vi "Day 12 Task 1 no recurse.vi"() -> ()   [LabVIEW 2018]
uses:
  Cave Info1.ctl
  <userlib>/_OpenG.lib/array/array.llb/Remove Duplicates from 1D Array (String)__ogtk.vi
  <userlib>/_OpenG.lib/array/array.llb/Search 1D Array (String)__ogtk.vi
panel:
  out "size(s)":i32
  out "Valid paths found":cluster{"Path":string[]}[](array[cluster])
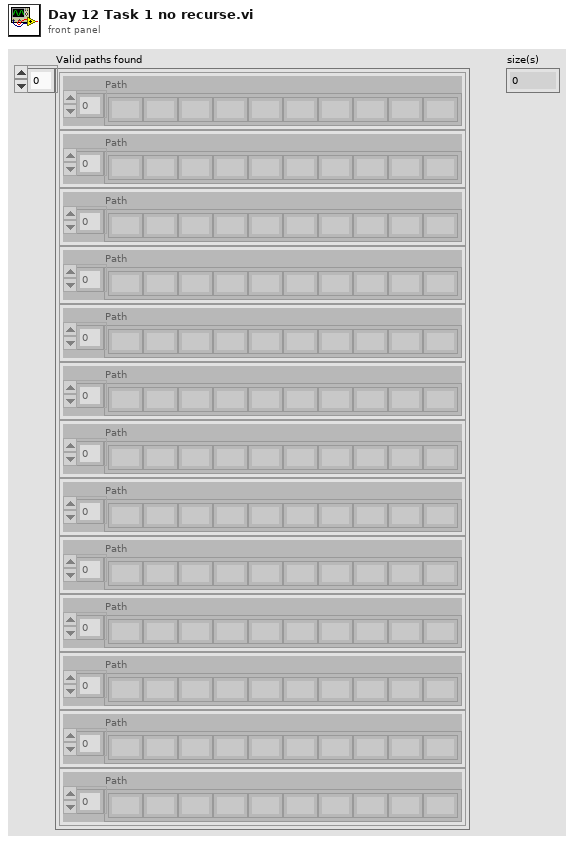
[diagram p1: front panel]
types:
  T1 = typedef "Cave Info1.ctl" = cluster{"Cave":string, "Is small?":bool, "Connections":string[]}
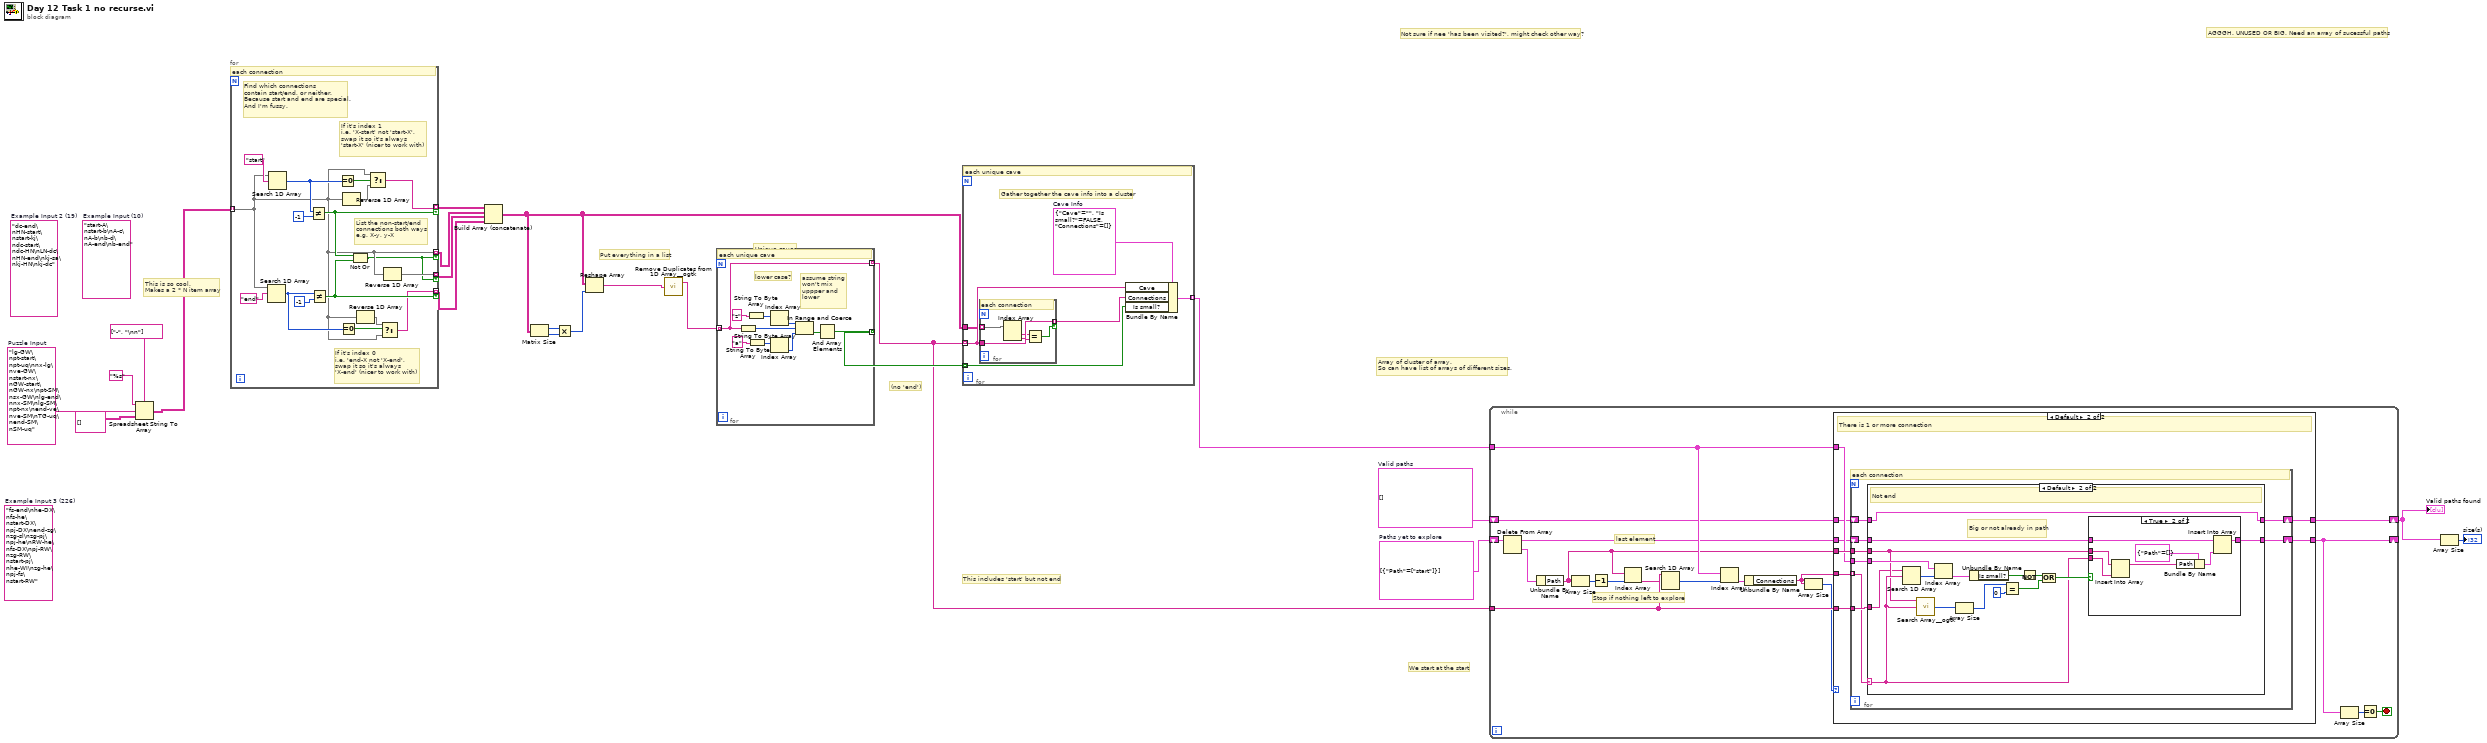
[diagram p0: block diagram]
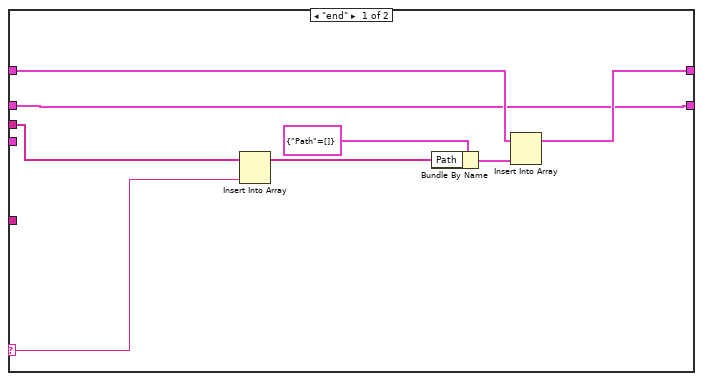
[diagram p3: hidden frame]
diagram:
  w7 = cluster{"Path":string[]}[] []  # Valid paths
  w9 = cluster{"Path":string[]}[] [{"Path"=["start"]}]  # Paths yet to explore
  (unwired) "fs-end\nhe-DX\nfs-he\nstart-DX\npj-DX\nend-zg\nzg-sl\nzg-pj\npj-he\nRW-he\nfs-DX\npj-RW\nzg-RW\nstart-pj\nhe-WI\nzg-he\npj-fs\nstart-RW"  # Example Input 3 (226)
  (unwired) "dc-end\nHN-start\nstart-kj\ndc-start\ndc-HN\nLN-dc\nHN-end\nkj-sa\nkj-HN\nkj-dc"  # Example Input 2 (19)
  w1 = "lg-GW\npt-start\npt-uq\nnx-lg\nve-GW\nstart-nx\nGW-start\nGW-nx\npt-SM\nsx-GW\nlg-end\nnx-SM\nlg-SM\npt-nx\nend-ve\nve-SM\nTG-uq\nend-SM\nSM-uq"  # Puzzle Input
  (unwired) "start-A\nstart-b\nA-c\nA-b\nb-d\nA-end\nb-end"  # Example Input (10)
  # "(no 'end')"
  # "We start at the start"
  # "Put everything in a list"
  # "Array of cluster of array.\nSo can have list of arrays of different sizes."
  # "AGGGH. UNUSED OR BIG. Need an array of sucessful paths"
  # "Not sure if nee 'has been visited?', might check other way?"
  # "This includes 'start' but not end"
  # "Unique caves"
  # "This is so cool.\nMakes a 2 * N item array"
  n1 = Spreadsheet String To Array(delimiter (Tab)=string[] ["-", "\nn"], format string="%s", spreadsheet string=w1, array type (2D Dbl)=string[][] []) -> (array=w15:string[][])
  n2 = for {
    tunnel: w15 -> [w25] mode=indexing
    tunnel: [w30] -> w14 mode=indexing if=w35
    tunnel: [w27] -> w11 mode=indexing if=w34
    tunnel: [w25] -> w13 mode=indexing if=w23
    tunnel: [w24] -> w12 mode=indexing if=w23
    # "List the non-start/end\nconnections both ways\ne.g. X-y, y-X"
    # "If it's index 0\ni.e. 'end-X not 'X-end',\nswap it so it's always \n'X-end' (nicer to work with)"
    # "Find which connections\ncontain start/end, or neither.\nBecause start and end are special.\nAnd I'm fussy."
    # "If it's index 1\ni.e. 'X-start' not 'start-X',\nswap it so it's always \n'start-X' (nicer to work with)"
    # "each connection"
    n3 = Search 1D Array(1D array=w25, element="end") -> (index of element=w26:i32)  [unwired: 1 in]
    n4 = Search 1D Array(1D array=w25, element="start") -> (index of element=w33:i32)  [unwired: 1 in]
    n5 = Not Equal?(x=w33, y=-1) -> (x != y?=w35:bool)
    n6 = Not Equal?(x=w26, y=-1) -> (x != y?=w34:bool)
    n7 = Equal To 0?(x=w33) -> (x = 0?=w32:bool)
    n8 = Equal To 0?(x=w26) -> (x = 0?=w29:bool)
    n9 = Reverse 1D Array(array=w25) -> (reversed array=w31:string[])
    n10 = Not Or(1:w34, 2:w35) -> (0:w23:bool)
    n11 = Reverse 1D Array(array=w25) -> (reversed array=w28:string[])
    n12 = Select(t=w25, s=w32, f=w31) -> (s? t:f=w30:string[])
    n13 = Select(t=w28, s=w29, f=w25) -> (s? t:f=w27:string[])
    n14 = Reverse 1D Array(array=w25) -> (reversed array=w24:string[])
  }
  n15 = Build Array (concatenate)(w14, w13, w12, w11) -> (w4:string[][])
  n16 = Matrix Size(0:w4) -> (1:w18:i32, 2:w19:i32)
  n17 = Multiply(x=w18, y=w19) -> (x*y=w17:i32)
  n18 = Reshape Array(w4, w17) -> (w16:string[])
  n19 = call-poly <userlib>:"Remove Duplicates from 1D Array__ogtk.vi"("Input Array"=w16) -> ("Output Array"=w3:string[])  [unwired: 1 out]
  n20 = for {
    tunnel: w3 -> [w40] mode=indexing
    tunnel: [w40] -> w2 mode=indexing
    tunnel: [w41] -> w10 mode=indexing
    # "lower case?"
    # "assume string \nwon't mix\nuppper and\nlower"
    # "each unique cave"
    n21 = String To Byte Array(string=w40) -> (unsigned byte array=w49:u8[])
    n22 = String To Byte Array(string="z" ("format string")) -> (unsigned byte array=w47:u8[])
    n23 = String To Byte Array(string="a" ("format string")) -> (unsigned byte array=w45:u8[])
    n24 = Index Array(array=w47) -> (element=w46:u8)  [unwired: 1 in]
    n25 = Index Array(array=w45) -> (element=w43:u8)  [unwired: 1 in]
    n26 = In Range and Coerce(upper limit=w46, x=w49, lower limit=w43) -> (In Range?=w42:bool[])  [unwired: 1 out]
    n27 = And Array Elements(Boolean array=w42) -> (logical AND=w41:bool)
  }
  n28 = for {
    tunnel: w2 -> [w54] mode=indexing
    tunnel: w4 -> [w51]
    tunnel: [w52] -> w8 mode=indexing
    tunnel: w10 -> [w50] mode=indexing
    w55 = T1 {"Cave"="", "Is small?"=FALSE, "Connections"=[]}  # Cave Info
    # "Gather together the cave info into a cluster"
    # "each unique cave"
    n29 = for {
      tunnel: w54 -> [w60]
      tunnel: [w58] -> w53 mode=indexing if=w59
      tunnel: w51 -> [w56] mode=indexing
      # "each connection"
      n30 = Index Array(array=w56) -> (element #1=w57:string, element #2=w58:string)  [unwired: 2 in]
      n31 = Equal?(x=w57, y=w60) -> (x = y?=w59:bool)
    }
    n32 = Bundle By Name(cluster=w55, "Cave"=w54, "Connections"=w53, "Is small?"=w50) -> (w52:T1)
  }
  n33 = while {
    tunnel: w2 -> [w76]
    tunnel: w8 -> [w75]
    shift-right: [w62] -> _
    shift-left: w9 -> [w65]
    shift-right: [w61] -> w6
    shift-left: w7 -> [w74]
    stop <- w78 stop-if-true
    # "last element"
    # "Stop if nothing left to explore"
    n34 = Delete From Array(array=w65) -> (deleted portion=w64:cluster{"Path":string[]}, array with subset deleted=w63:cluster{"Path":string[]}[])  [unwired: 2 in]
    n35 = Unbundle By Name(w64) -> ("Path"=w68:string[])
    n36 = Array Size(array=w68) -> (size(s)=w73:i32)
    n37 = Decrement(x=w73) -> (x-1=w72:i32)
    n38 = Index Array(array=w68, index=w72) -> (element=w71:string)
    n39 = Search 1D Array(1D array=w76, element=w71) -> (index of element=w70:i32)  [unwired: 1 in]
    n40 = Index Array(array=w75, index=w70) -> (element=w69:T1)
    n41 = Unbundle By Name(w69) -> ("Connections"=w67:string[])
    n42 = Array Size(array=w67) -> (size(s)=w66:i32)
    n43 = case shown="Default" w66 {
      tunnel: w68 -> [_ w88]
      tunnel: w76 -> [_ w87]
      tunnel: w75 -> [_ w86]
      tunnel: w74 -> [w80 w85]
      tunnel: [w80 w84] -> w61
      tunnel: w67 -> [_ w83]
      tunnel: w63 -> [w79 w82]
      tunnel: [w79 w81] -> w62
      frame 0 {
        # "No more connections,\nlet it unqueue the next thing"
      }
      frame Default {
        # "There is 1 or more connection"
        n44 = for {
          tunnel: w83 -> [w93] mode=indexing
          tunnel: w88 -> [w96]
          tunnel: w87 -> [w95]
          tunnel: w86 -> [w94]
          shift-right: [w91] -> w84
          shift-left: w85 -> [w92]
          shift-right: [w89] -> w81
          shift-left: w82 -> [w90]
          # "each connection"
          n45 = case shown="Default" w93 {
            selector: w93 -> [w104 w108]
            tunnel: w96 -> [w98 w107]
            tunnel: w95 -> [_ w106]
            tunnel: w94 -> [_ w119]
            tunnel: w92 -> [w103 w117]
            tunnel: [w99 w117] -> w91
            tunnel: w90 -> [w97 w113]
            tunnel: [w97 w112] -> w89
            frame "end" {
              n46 = Insert Into Array(array=w98, new element=w104) -> (w101:string[])  [unwired: 1 in]
              n47 = Bundle By Name(cluster=cluster{"Path":string[]} {"Path"=[]} ("new element/subarray"), "Path"=w101) -> (w100:cluster{"Path":string[]})
              n48 = Insert Into Array(array=w103, new element=w100) -> (w99:cluster{"Path":string[]}[])  [unwired: 1 in]
            }
            frame Default {
              # "Big or not already in path"
              # "Not end"
              n49 = Search 1D Array(1D array=w106, element=w108) -> (index of element=w120:i32)  [unwired: 1 in]
              n50 = call-poly <userlib>:"Search Array__ogtk.vi"("Array"=w107, "Element Data"=w108) -> ("Indices of Elements"=w109:i32[])  [unwired: 7 in]
              n51 = Index Array(array=w119, index=w120) -> (element=w118:T1)
              n52 = Array Size(array=w109) -> (size(s)=w105:i32)
              n53 = Unbundle By Name(w118) -> ("Is small?"=w116:bool)
              n54 = Equal?(x=w105, y=0) -> (x = y?=w114:bool)
              n55 = Not(x=w116) -> (.not. x?=w115:bool)
              n56 = Compound Arithmetic op=OR(w115, w114) -> (w111:bool)
              n57 = case shown="True" w111 {
                tunnel: w107 -> [_ w126]
                tunnel: w108 -> [_ w125]
                tunnel: w113 -> [w121 w124]
                tunnel: [w121 w123] -> w112
                frame False {
                }
                frame True {
                  n58 = Insert Into Array(array=w126, new element=w125) -> (w127:string[])  [unwired: 1 in]
                  n59 = Bundle By Name(cluster=cluster{"Path":string[]} {"Path"=[]} ("new element/subarray"), "Path"=w127) -> (w122:cluster{"Path":string[]})
                  n60 = Insert Into Array(array=w124, new element=w122) -> (w123:cluster{"Path":string[]}[])  [unwired: 1 in]
                }
              }
            }
          }
        }
      }
    }
    n61 = Array Size(array=w62) -> (size(s)=w77:i32)
    n62 = Equal To 0?(x=w77) -> (x = 0?=w78:bool)
  }
  "Valid paths found" <- w6
  n63 = Array Size(array=w6) -> (size(s)=→"size(s)":i32)
